vi "for_v0_v2.vi"() -> ()   [LabVIEW 2010]
panel:
  out "Numeric":dbl
  out "Array":bool[](array[boolean])=[FALSE, TRUE, FALSE, FALSE, TRUE, FALSE, TRUE, TRUE]
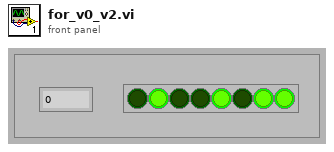
[diagram p1: front panel]
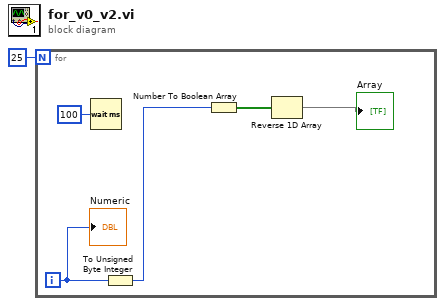
[diagram p0: block diagram]
diagram:
  n1 = for {
    N: 25 -> [_]
    i -> [w2]
    n2 = Wait (ms)(milliseconds to wait=u32 100) -> ()  [unwired: 1 out]
    n3 = To Unsigned Byte Integer(number=w2) -> (unsigned 8bit integer=w3:u8)
    n4 = Number To Boolean Array(number=w3) -> (Boolean array=w6:bool[])
    n5 = Reverse 1D Array(array=w6) -> (reversed array=→"Array":bool[])
    "Numeric" <- w2
  }
